vi "Configure Library for Build.vi"(9 "enable debug? (F)":bool, 11 "library path":path) -> (0 "error out":errorcluster)   [LabVIEW 2017, in "Build Automation.lvlib"]
uses:
  Build Automation.lvlib
  <vilib>/Utility/EditLVProj/Edit LVProj.lvlib
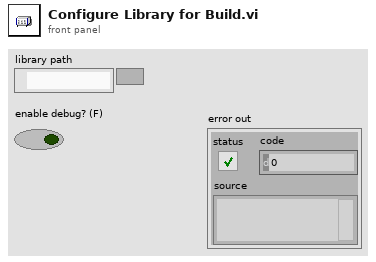
[diagram p1: front panel]
types:
  T1 = enum16{"Share clones between instances", "Preallocate clone for each instance"}
  T2 = cluster{"Status Message":refnum<data-value>, "Progress":refnum<data-value>, "Stop":refnum<data-value>}
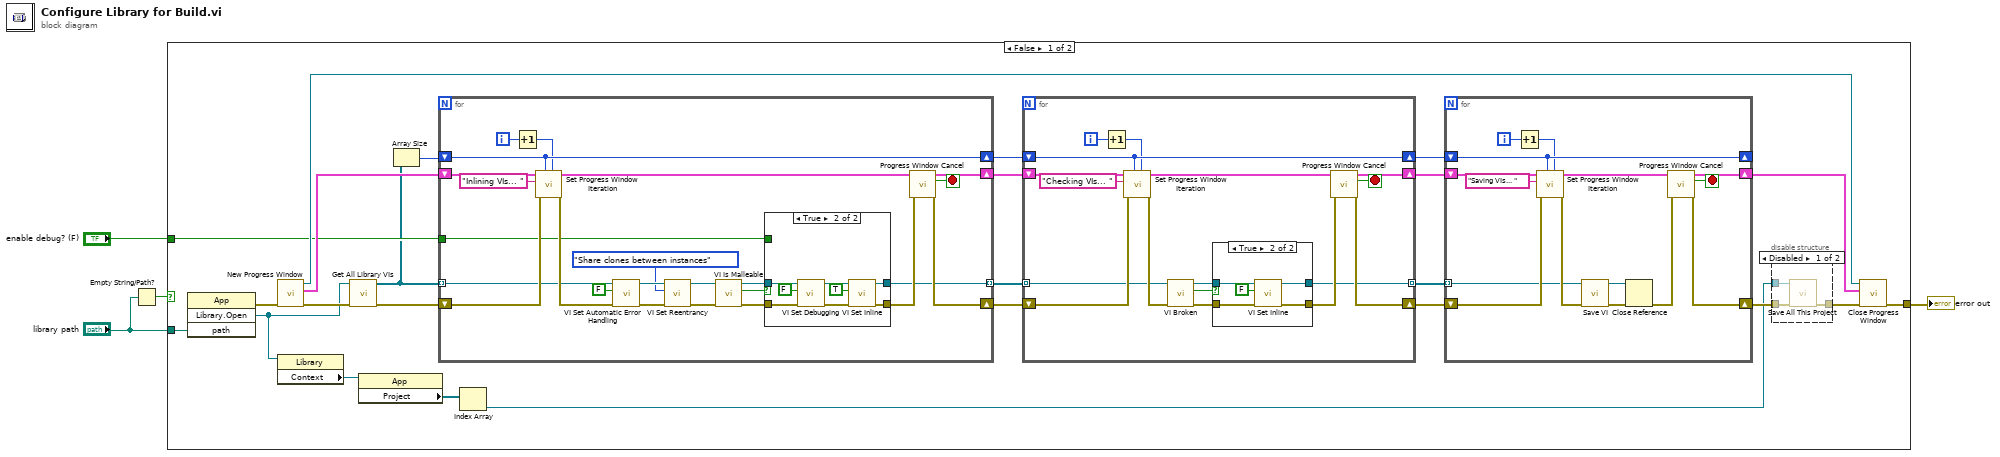
[diagram p0: block diagram]
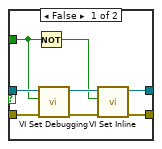
[diagram p3: hidden frame]
diagram:
  n1 = Empty String/Path?(string/path="library path") -> (empty?=w1:bool)
  n2 = case shown="False" w1 {
    tunnel: [w24 _] -> w4
    tunnel: "enable debug? (F)" -> [w23 _]
    tunnel: "library path" -> [w5 _]
    frame False {
      n3 = invoke class="App" method="Library.Open"("path"=w5) -> (error out=w28:errorcluster, "Open Library"=w16:refnum<vi>)  [unwired: 3 in, 2 out]
      n4 = call "New Progress Window.vi"("error in (no error)"=w28) -> ("error out"=w26:errorcluster, "DVRs"=w25:T2, "VI refnum"=w27:refnum<vi>)  [unwired: 8 in]
      n5 = property class="Library"(reference=w16) -> ("Context"=w15:refnum<vi>)  [unwired: 1 in, 2 out]
      n6 = call "Get All Library VIs.vi"("error in (no error)"=w26, "library ref"=w16) -> ("error out"=w29:errorcluster, "vi refs"=w21:refnum<vi>[])  [unwired: 8 in]
      n7 = property class="App"(reference=w15) -> ("Project"=w14:refnum<vi>[])  [unwired: 1 in, 2 out]
      n8 = Array Size(array=w21) -> (size(s)=w22:i32)
      n9 = for {
        tunnel: w21 -> [w40] mode=indexing
        shift-right: [w55] -> w19
        shift-left: w25 -> [w45]
        shift-right: [w41] -> w17
        shift-left: w29 -> [w43]
        tunnel: w23 -> [w39]
        tunnel: [w34] -> w18 mode=indexing
        shift-right: [w38] -> w20
        shift-left: w22 -> [w38]
        i -> [w57]
        stop <- w56 stop-if-true
        n10 = Increment(x=w57) -> (x+1=w37:i32)
        n11 = call "Set Progress Window Iteration.vi"("current iteration"=w37, "total iterations"=w38, "error in (no error)"=w43, "Status Message"="Inlining VIs... ", "DVRs in"=w45) -> ("error out"=w42:errorcluster, "DVRs out"=w44:T2)  [unwired: 5 in]
        n12 = call "VI Set Automatic Error Handling.vi"("error in (no error)"=w42, "Automatic Error Handling"=FALSE, "vi ref in"=w40) -> ("error out"=w52:errorcluster, "vi ref out"=w53:refnum<vi>)  [unwired: 7 in]
        n13 = call "VI Set Reentrancy.vi"("error in (no error)"=w52, "Reentrancy Type"=T1."Share clones between instances", "vi ref in"=w53) -> ("error out"=w49:errorcluster, "vi ref out"=w50:refnum<vi>)  [unwired: 7 in]
        n14 = call "VI Is Malleable.vi"("error in (no error)"=w49, "vi ref in"=w50) -> ("error out"=w48:errorcluster, "malleable VI?"=w46:bool, "vi ref out"=w47:refnum<vi>)  [unwired: 7 in]
        n15 = case shown="True" w46 {
          tunnel: [w63 w71] -> w34
          tunnel: [w62 w70] -> w35
          tunnel: w48 -> [w59 w68]
          tunnel: w47 -> [w60 w69]
          tunnel: w39 -> [w58 _]
          frame False {
            n16 = Not(x=w58) -> (.not. x?=w61:bool)
            n17 = call "VI Set Debugging.vi"("error in (no error)"=w59, "Allow Debugging"=w58, "vi ref in"=w60) -> ("error out"=w64:errorcluster, "vi ref out"=w65:refnum<vi>)  [unwired: 7 in]
            n18 = call "VI Set Inline.vi"("error in (no error)"=w64, "Inline VI"=w61, "vi ref in"=w65) -> ("error out"=w62:errorcluster, "vi ref out"=w63:refnum<vi>)  [unwired: 7 in]
          }
          frame True {
            n19 = call "VI Set Debugging.vi"("error in (no error)"=w68, "Allow Debugging"=FALSE, "vi ref in"=w69) -> ("error out"=w72:errorcluster, "vi ref out"=w73:refnum<vi>)  [unwired: 7 in]
            n20 = call "VI Set Inline.vi"("error in (no error)"=w72, "Inline VI"=TRUE, "vi ref in"=w73) -> ("error out"=w70:errorcluster, "vi ref out"=w71:refnum<vi>)  [unwired: 7 in]
          }
        }
        n21 = call "Progress Window Cancel.vi"("error in (no error)"=w35, "DVRs in"=w44) -> ("error out"=w41:errorcluster, "cancelled"=w56:bool, "DVRs out"=w55:T2)  [unwired: 7 in]
      }
      n22 = Index Array(array=w14) -> (element=w7:refnum<vi>)  [unwired: 1 in]
      n23 = for {
        tunnel: w18 -> [w79] mode=indexing
        shift-right: [w88] -> w12
        shift-left: w19 -> [w87]
        shift-right: [w84] -> w10
        shift-left: w17 -> [w85]
        shift-right: [w83] -> w11
        shift-left: w20 -> [w83]
        tunnel: [w74] -> w9 mode=indexing
        i -> [w90]
        stop <- w89 stop-if-true
        n24 = Increment(x=w90) -> (x+1=w82:i32)
        n25 = call "Set Progress Window Iteration.vi"("current iteration"=w82, "total iterations"=w83, "error in (no error)"=w85, "Status Message"="Checking VIs... ", "DVRs in"=w87) -> ("error out"=w80:errorcluster, "DVRs out"=w86:T2)  [unwired: 5 in]
        n26 = call "VI Broken.vi"("error in (no error)"=w80, "vi ref in"=w79) -> ("error out"=w77:errorcluster, "broken?"=w76:bool, "vi ref out"=w78:refnum<vi>)  [unwired: 7 in]
        n27 = case shown="True" w76 {
          tunnel: [w92 w97] -> w74
          tunnel: [w91 w96] -> w75
          tunnel: w77 -> [w91 w95]
          tunnel: w78 -> [w92 w93]
          frame False {
          }
          frame True {
            n28 = call "VI Set Inline.vi"("error in (no error)"=w95, "Inline VI"=FALSE, "vi ref in"=w93) -> ("error out"=w96:errorcluster, "vi ref out"=w97:refnum<vi>)  [unwired: 7 in]
          }
        }
        n29 = call "Progress Window Cancel.vi"("error in (no error)"=w75, "DVRs in"=w86) -> ("error out"=w84:errorcluster, "cancelled"=w89:bool, "DVRs out"=w88:T2)  [unwired: 7 in]
      }
      n30 = for {
        tunnel: w9 -> [w98] mode=indexing
        shift-right: [w110] -> w6
        shift-left: w12 -> [w109]
        shift-right: [w106] -> w8
        shift-left: w10 -> [w107]
        shift-right: [w105] -> _
        shift-left: w11 -> [w105]
        i -> [w112]
        stop <- w111 stop-if-true
        n31 = Increment(x=w112) -> (x+1=w104:i32)
        n32 = call "Set Progress Window Iteration.vi"("current iteration"=w104, "total iterations"=w105, "error in (no error)"=w107, "Status Message"="Saving VIs... ", "DVRs in"=w109) -> ("error out"=w102:errorcluster, "DVRs out"=w108:T2)  [unwired: 5 in]
        n33 = call "Save VI.vi"("error in (no error)"=w102, "vi ref in"=w98) -> ("error out"=w100:errorcluster, "vi ref out"=w101:refnum<vi>)  [unwired: 8 in]
        n34 = Close Reference(reference=w101, error in (no error)=w100) -> (error out=w99:errorcluster)
        n35 = call "Progress Window Cancel.vi"("error in (no error)"=w99, "DVRs in"=w108) -> ("error out"=w106:errorcluster, "cancelled"=w111:bool, "DVRs out"=w110:T2)  [unwired: 7 in]
      }
      n36 = disable-structure shown="Disabled" {
        disable-tunnel: [w32 w33] -> w13
        disable-tunnel: w8 -> [w31 w33]
        disable-tunnel: w7 -> [w30 _]
        frame Disabled {
          n37 = call <vilib>:"Save All This Project.vi"("error in (no error)"=w31, "Project in"=w30) -> ("error out"=w32:errorcluster)  [unwired: 8 in, 1 out]
        }
        frame Enabled {
        }
      }
      n38 = call "Close Progress Window.vi"("error in (no error)"=w13, "DVRs in"=w6, "VI refnum"=w27) -> ("error out"=w24:errorcluster)  [unwired: 8 in]
    }
    frame True {
    }
  }
  "error out" <- w4
